vi "Start Discovery.vi"() -> (4 "VI Path":path, 8 "user events":T1, 15 "error out":errorcluster)   [LabVIEW 2020, in "epl-network.lvlib"]
uses:
  epl-network.lvlib
  Private/Discovered Host.ctl
  Typedefs/Server Beacon.ctl
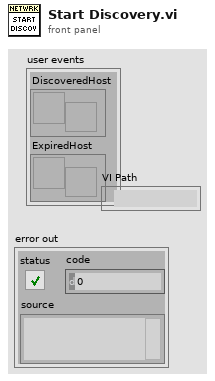
[diagram p1: front panel]
types:
  T1 = cluster{"DiscoveredHost":refnum<user-event>, "ExpiredHost":refnum<user-event>}
  T2 = typedef "epl-network.lvlib/Discovered Host.ctl" = cluster{"Beacon":T3, "Last Seen":timestamp}
  T3 = typedef "epl-network.lvlib/Server Beacon.ctl" = cluster{"name":string, "addr":string, "port":u16, "ver":u16}
  T4 = cluster{refnum<vi>, "notifier out":refnum<notifier>, cluster{"DiscoveredHost":refnum<user-event>, "ExpiredHost":refnum<user-event>}}
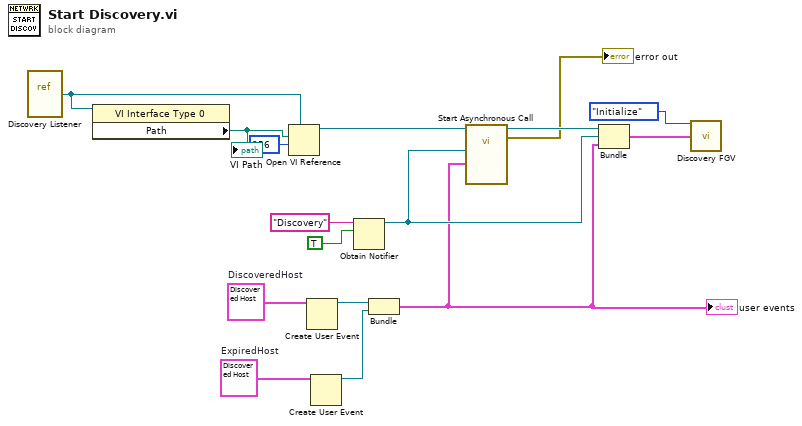
[diagram p0: block diagram]
diagram:
  w13 = T2 {"Beacon"={"name"="", "addr"="", "port"=0, "ver"=10001}, "Last Seen"=timestamp(0 s since 1904-01-01)}  # ExpiredHost
  w14 = T2 {"Beacon"={"name"="", "addr"="", "port"=0, "ver"=10001}, "Last Seen"=timestamp(0 s since 1904-01-01)}  # DiscoveredHost
  n1 = vi-ref "Discovery Listener.vi"() -> (w1:refnum<vi>)
  n2 = property class="VI Interface Type 0"(reference=w1) -> ("Path"=w2:path)  [unwired: 1 in, 2 out]
  "VI Path" <- w2
  n3 = Open VI Reference(type specifier VI Refnum (for type only)=w1, vi path=w2, options=256) -> (vi reference=w3:refnum<vi>)  [unwired: 3 in, 1 out]
  n4 = Create User Event(user event datatype=w14) -> (user event=w12:refnum<user-event>)  [unwired: 1 in, 1 out]
  n5 = Create User Event(user event datatype=w13) -> (user event=w11:refnum<user-event>)  [unwired: 1 in, 1 out]
  n6 = Obtain Notifier(name (unnamed)="Discovery", notification data type=TRUE) -> (notifier out=w9:refnum<notifier>)  [unwired: 2 in, 2 out]
  n7 = Bundle("DiscoveredHost"=w12, "ExpiredHost"=w11) -> (w8:T1)  [unwired: 1 in]
  "user events" <- w8
  n8 = call-by-ref "Start Asynchronous Call"(reference=w3, "stop notifier"=w9, "Discovery Events"=w8) -> (reference out=w10:refnum<vi>, error out=→"error out":errorcluster)  [unwired: 14 in, 1 out]
  n9 = Bundle(w10, "notifier out"=w9, w8) -> (w7:T4)  [unwired: 1 in]
  n10 = call "Discovery FGV.vi"("action"=enum16{"Initialize", "Get"}."Initialize", "data in"=w7) -> ()  [unwired: 13 in, 1 out]
